vi "AmmeterGlobalCostants.vi"() -> ()   [LabVIEW 2010]
uses:
  types/VarableStruct.ctl
  types/VarableID.ctl
panel:
  in  "AppLayerCmd":refnum<k20>
  in  "StorageFileRef":refnum<file>
  in  "displayRefs":T1
  in  "SerialPort2":refnum<visa-resource-name>="COM9"
  in  "SerialPort1":refnum<visa-resource-name>="COM7"
  out "EXIT":bool
  in  "PortIPList 2":string[](array[string])
  in  "PortIPList":string[](array[string])
  in  "CommandCodeList":cluster{"CommandCode":string, "VarableID":T2}[](array[cluster])=[{"CommandCode"="68####68110435353433", "VarableID"=enum."current"}, {"CommandCode"="68####68110433343435", "VarableID"=enum."voltage"}, {"CommandCode"="68####68110435383433", "VarableID"=enum."power"}, {"CommandCode"="68####68110435393433", "VarableID"=enum."PF"}]
  in  "VarableList":T3[](array[typedef])
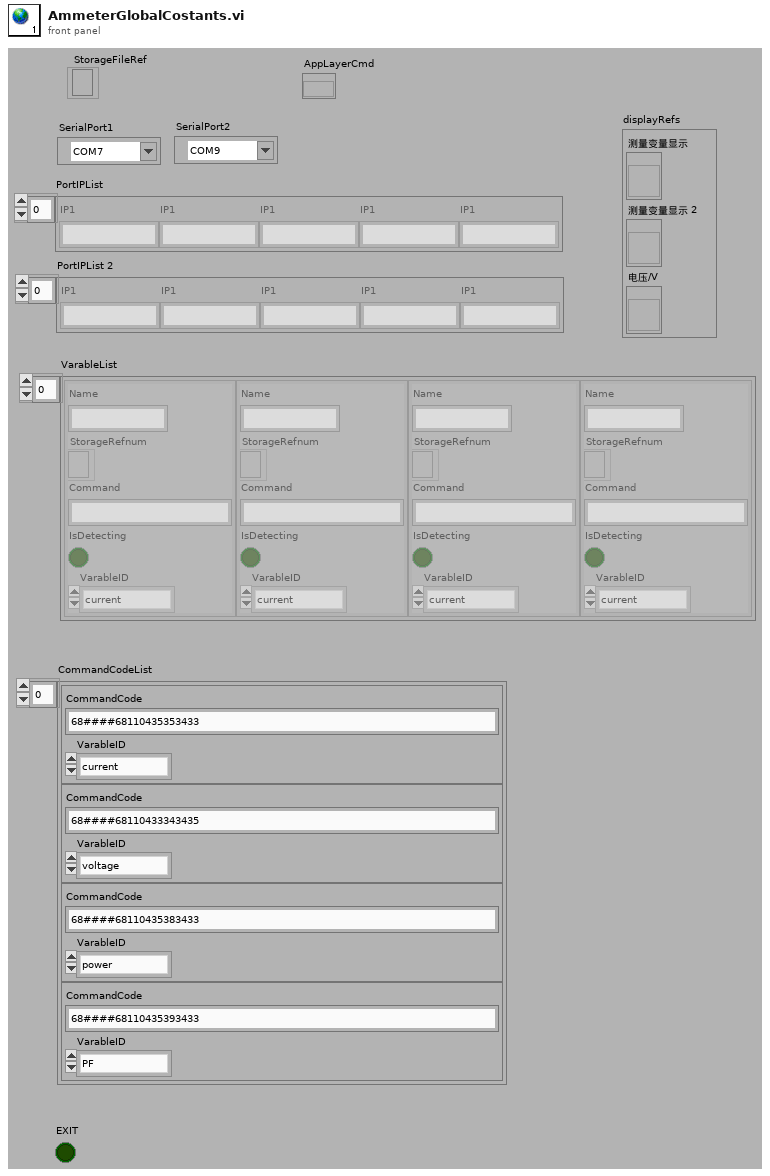
[diagram p1: front panel]
types:
  T1 = cluster{"测量变量显示":refnum<vi>, "测量变量显示 2":refnum<vi>, "电压/V":refnum<vi>}
  T2 = typedef "VarableID.ctl" = enum16{"current", "power", "PF", "voltage"}
  T3 = typedef "VarableStruct.ctl" = cluster{"Name":string, "StorageRefnum":refnum<file>, "Command":string, "IsDetecting":bool, "VarableID":T2}
diagram:
